vi "multinumericlimittest1.vi"(4 "Sequence Context":refnum<k7>) -> (0 "error out":errorcluster)   [LabVIEW 2011]
doc: "Simulates measuring four values, then sets the step results using the TestStand Utility functions."
uses:
  <vilib>/addons/TestStand/_TSUtility.llb/TestStand - Set Property Value (Numeric Array).vi
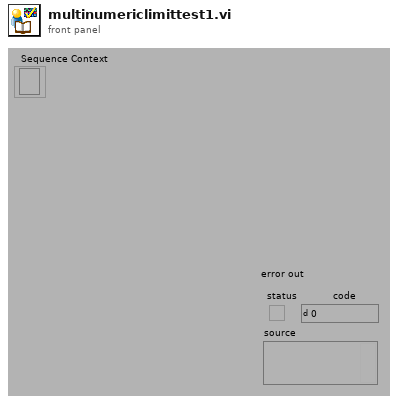
[diagram p1: front panel]
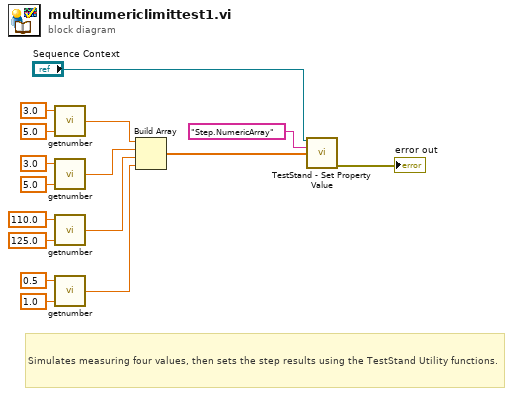
[diagram p0: block diagram]
diagram:
  # "Simulates measuring four values, then sets the step results using the TestStand Utility functions."
  n1 = call "getnumber.vi"("High Limit"=5.0, "Low Limit"=3.0) -> ("Random Number within Limits"=w3:dbl)  [unwired: 3 out]
  n2 = call "getnumber.vi"("High Limit"=5.0, "Low Limit"=3.0) -> ("Random Number within Limits"=w4:dbl)  [unwired: 3 out]
  n3 = call "getnumber.vi"("High Limit"=125.0, "Low Limit"=110.0) -> ("Random Number within Limits"=w5:dbl)  [unwired: 3 out]
  n4 = call "getnumber.vi"("High Limit"=1.0, "Low Limit"=0.5) -> ("Random Number within Limits"=w6:dbl)  [unwired: 3 out]
  n5 = Build Array(w3, w4, w5, w6) -> (w2:dbl[])
  n6 = call-poly <vilib>:"TestStand - Set Property Value.vi"("Sequence Context In"="Sequence Context", "Lookup String"="Step.NumericArray", "New Value"=w2) -> ("error out"=→"error out":errorcluster)  [unwired: 2 in, 10 out]
